vi "H-bridge and gear motor_0.vi"() -> ()   [LabVIEW 2015]
uses:
  <vilib>/myRIO/Common/Instrument Driver Framework/myRIO v1.0/Encoder/typedefs/Encoder Count Direction Enum.ctl
  <vilib>/myRIO/Instrument Drivers/Onboard IO/Encoder/vis/Read.vi
  <vilib>/myRIO/Instrument Drivers/Onboard IO/PWM/vis/Set Duty Cycle and Frequency.vi
  <vilib>/myRIO/Instrument Drivers/Onboard IO/DIO/vis/Write.vi
  <vilib>/myRIO/Common/Instrument Driver Framework/myRIO v1.0/UART/vis/myRIO v1.0 Close UART.vi
  <vilib>/myRIO/Instrument Drivers/Onboard IO/Encoder/vis/Smart Open.vi
  <vilib>/Utility/error.llb/Error Cluster From Error Code.vi
  <vilib>/myRIO/Common/Instrument Driver Framework/myRIO v1.0/Encoder/vis/myRIO v1.0 Read Encoder.vi
  <vilib>/myRIO/Instrument Drivers/Onboard IO/PWM/vis/Smart Open.vi
  <vilib>/myRIO/Common/Instrument Driver Framework/myRIO v1.0/PWM/vis/myRIO v1.0 Write PWM.vi
  <vilib>/myRIO/Instrument Drivers/Onboard IO/DIO/vis/Smart Open.vi
  <vilib>/myRIO/Common/Instrument Driver Framework/myRIO v1.0/DIO/vis/myRIO v1.0 Write DIO.vi
  <vilib>/myRIO/Common/Instrument Driver Framework/Utilities/vis/FPGA Ref Manager.vi
  <vilib>/myRIO/Common/Instrument Driver Framework/myRIO v1.0/myRIO v1.0 Reset FPGA.vi
  <vilib>/myRIO/Common/Instrument Driver Framework/myRIO v1.0/IRQ/vis/myRIO v1.0 IRQ Info FGV.vi
  <vilib>/myRIO/Common/Instrument Driver Framework/myRIO v1.0/IRQ/vis/myRIO v1.0 Timer IRQ Info FGV.vi
  <vilib>/myRIO/Common/Instrument Driver Framework/myRIO v1.0/IRQ/vis/myRIO v1.0 ISR Agent.vi
  <vilib>/myRIO/Instrument Drivers/Utilities/Utilities.lvlib
panel:
  in  "Tab Control":enum32{"Page 1", "Page 2"}(tab)
  in  "Reset Counter":bool
  out "Counter Direction":T1
  out "Counter Value":i32
  out "Direction":bool
  in  "Enable":bool
  in  "PWM duty  [%]":dbl(slide) scale=-100.0..100.0
  in  "[ESC]":bool
  # "Pardeep kumar"
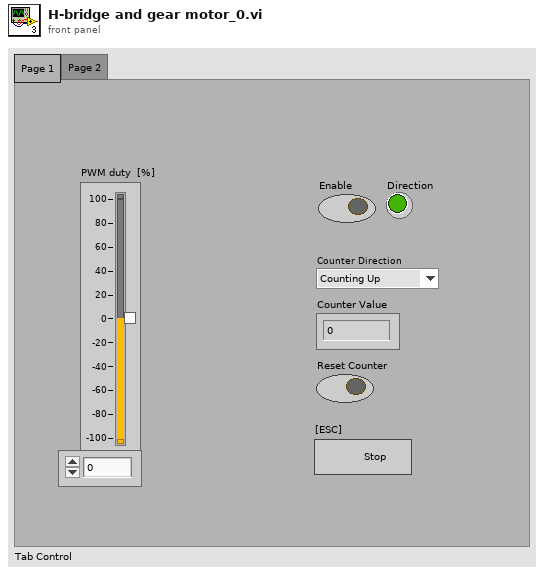
[diagram p1: front panel]
types:
  T1 = typedef "Encoder Count Direction Enum.ctl" = enum16{"Counting Up", "Counting Down"}
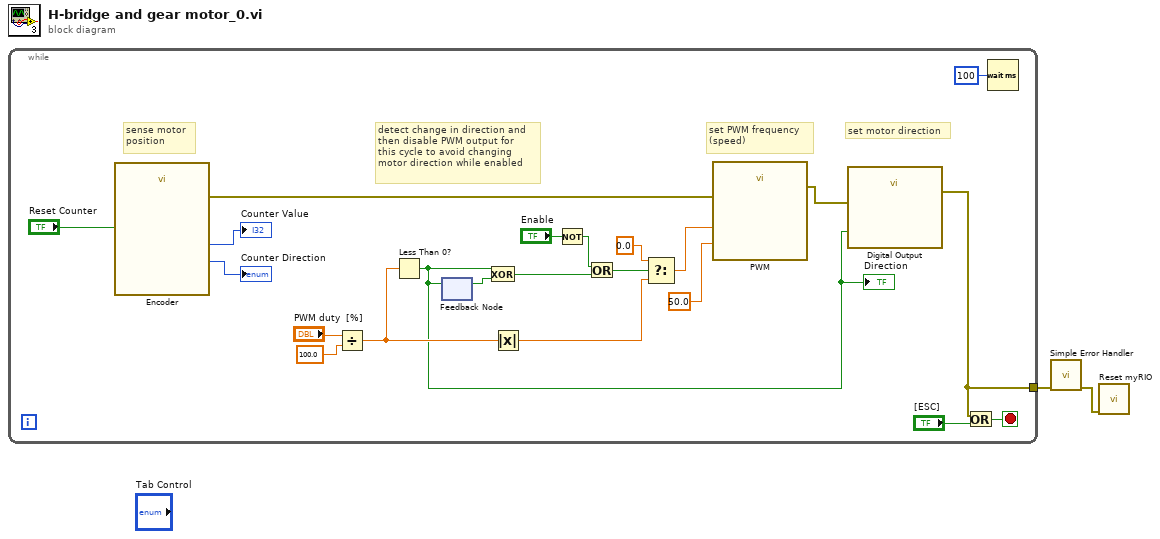
[diagram p0: block diagram]
diagram:
  n1 = while {
    tunnel: [w17] -> w1
    stop <- w24 stop-if-true
    # "sense motor \nposition"
    # "detect change in direction and\nthen disable PWM output for\nthis cycle to avoid changing\nmotor direction while enabled"
    # "set PWM frequency\n(speed)"
    # "set motor direction"
    n2 = call "Encoder"("Reset Counter"="Reset Counter") -> ("Counter Value"=→"Counter Value":i32, "Counter Direction"=→"Counter Direction":T1, "error out"=w21:errorcluster)  [unwired: 23 in, 1 out]
    n3 = Divide(x="PWM duty  [%]", y=100.0) -> (x/y=w9:dbl)
    n4 = Less Than 0?(x=w9) -> (x < 0?=w4:bool)
    "Direction" <- w4
    n5 = feedback-in #1(w4) -> ()
    n6 = feedback #1() -> (w19:bool)  [unwired: 1 in]
    n7 = Exclusive Or(1:w19, 2:w4) -> (0:w16:bool)
    n8 = Absolute Value(x=w9) -> (abs(x)=w6:dbl)
    n9 = Not(x="Enable") -> (.not. x?=w13:bool)
    n10 = Or(x=w13, y=w16) -> (x .or. y?=w15:bool)
    n11 = Select(t=0.0 ("f"), s=w15, f=w6) -> (s? t:f=w8:dbl)
    n12 = call "PWM"("Duty Cycle (0-1)"=w8, "Frequency (Hz)"=50.0, "error in (no error)"=w21) -> ("error out"=w20:errorcluster)  [unwired: 24 in]
    n13 = call "Digital Output"("A/DIO0 (Pin 11)"=w4, "error in (no error)"=w20) -> ("error out"=w17:errorcluster)  [unwired: 25 in]
    n14 = Or(x=w17, y="[ESC]") -> (x .or. y?=w24:bool)
    n15 = Wait (ms)(milliseconds to wait=u32 100) -> ()  [unwired: 1 out]
  }
  n16 = call <vilib>:"Simple Error Handler.vi"("error in (no error)"=w1) -> ("error out"=w2:errorcluster)  [unwired: 4 in, 4 out]
  n17 = call <vilib>:"Reset myRIO.vi"("error in (no error)"=w2) -> ()  [unwired: 10 in, 1 out]
